vi "Create.vi"(8 "error in (no error)":errorcluster, 10 "objects":refnum<class>[](array[class]), 11 "name":string) -> (0 "error out":errorcluster, 3 "Component":refnum<class "Component.lvclass">)   [LabVIEW 2017, in "DSF Core.lvlib" / "Component.lvclass"]
uses:
  Component.lvclass
  Component.lvclass/Component.ctl
  Component User Interface/Component User Interfaces.lvclass
  Component Configuration/Component Configurations.lvclass
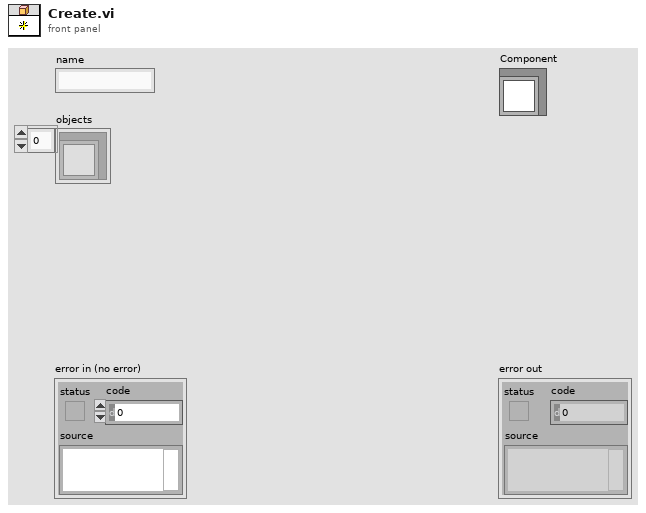
[diagram p1: front panel]
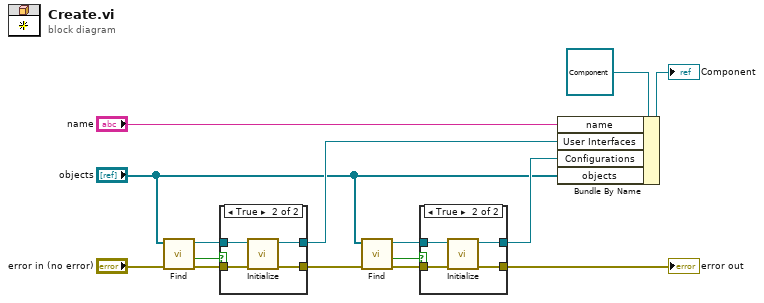
[diagram p0: block diagram]
diagram:
  n1 = call "Find.vi"("error in (no error)"="error in (no error)", "objects"="objects") -> ("error out"=w10:errorcluster, "found?"=w11:bool, "Component User Interfaces"=w9:refnum<class "Component User Interfaces.lvclass">)  [unwired: 6 in, 1 out]
  n2 = case shown="True" w11 {
    tunnel: w10 -> [w16 w21]
    tunnel: w9 -> [w17 w20]
    tunnel: [w17 w19] -> w7
    tunnel: [w16 w18] -> w8
    frame False {
    }
    frame True {
      n3 = call-dynamic "Initialize.vi"("error in (no error)"=w21, "Component UI in"=w20) -> ("error out"=w18:errorcluster, "Component UI out"=w19:refnum<class "Component User Interfaces.lvclass">)  [unwired: 8 in]
    }
  }
  n4 = call "Find.vi"("error in (no error)"=w8, "objects"="objects") -> ("error out"=w6:errorcluster, "found?"=w4:bool, "Component Configurations"=w5:refnum<class "Component Configurations.lvclass">)  [unwired: 6 in, 1 out]
  n5 = case shown="True" w4 {
    tunnel: w6 -> [w22 w27]
    tunnel: w5 -> [w23 w26]
    tunnel: [w23 w24] -> w3
    tunnel: [w22 w25] -> w1
    frame False {
    }
    frame True {
      n6 = call-dynamic "Initialize.vi"("error in (no error)"=w27, "Component Configuration in"=w26) -> ("error out"=w25:errorcluster, "Component Configuration out"=w24:refnum<class "Component Configurations.lvclass">)  [unwired: 8 in]
    }
  }
  "error out" <- w1
  n7 = Bundle By Name(cluster=refnum<class "Component.lvclass"> refnum ("Component in"), "name"="name", "User Interfaces"=w7, "Configurations"=w3, "objects"="objects") -> (→"Component":refnum<class "Component.lvclass">)
